vi "UAMatchLabel.vi"(8 "error in (no error)":errorcluster caption="错误输入（无错误）", 11 "String":string) -> (0 "error out":errorcluster caption="错误输出", 3 "keyValues":T1(array[cluster]))   [LabVIEW 2014, in "OPCUA XML(dev).lvlib"]
uses:
  <vilib>/regexp/Match Regular Expression.xnode
  OPCUA XML(dev).lvlib
panel:
  out "Array":string[](array[string])
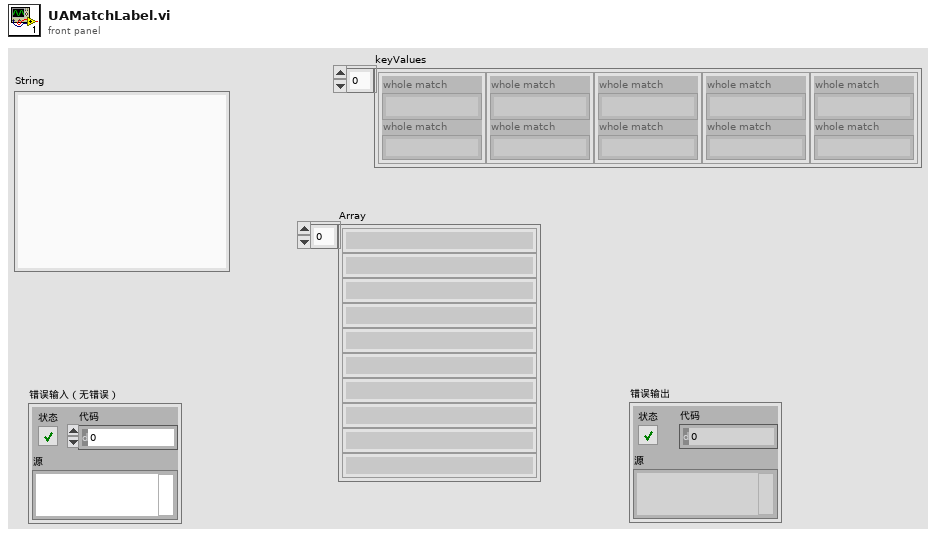
[diagram p1: front panel]
types:
  T1 = cluster{"whole match":string, "whole match":string}[]
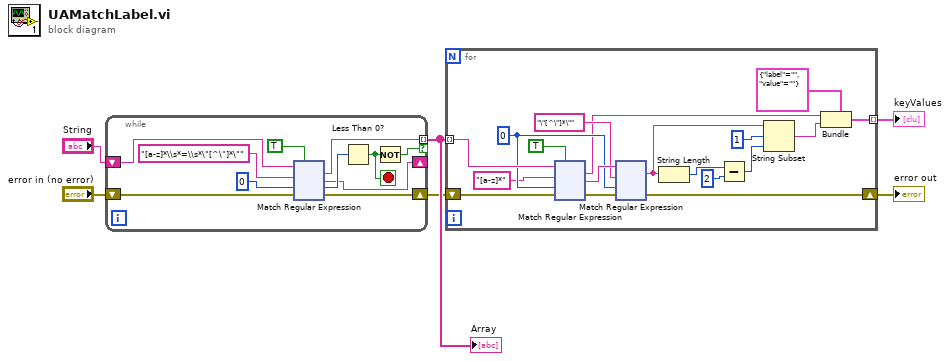
[diagram p0: block diagram]
diagram:
  n1 = while {
    shift-right: [w12] -> _
    shift-left: "String" -> [w17]
    tunnel: [w14] -> w4 mode=indexing if=w7
    shift-right: [w9] -> w3
    shift-left: "error in (no error)" -> [w10]
    stop <- w8 stop-if-true
    n2 = xnode "Match Regular Expression"("input string"=w17, "regular expression"="[a-z]*\\s*=\\s*\"[^\"]*\"", "offset (0)"=0, "error in"=w10, "ignore case? (F)"=TRUE) -> ("whole match"=w14:string, "after match"=w12:string, "offset past match"=w13:i32, "error out"=w9:errorcluster)  [unwired: 1 in, 1 out]
    n3 = Less Than 0?(x=w13) -> (x < 0?=w8:bool)
    n4 = Not(x=w8) -> (.not. x?=w7:bool)
  }
  "Array" <- w4
  n5 = for {
    tunnel: w4 -> [w149] mode=indexing
    shift-right: [w141] -> w2
    shift-left: w3 -> [w143]
    tunnel: [w133] -> w1 mode=indexing
    w145 = 0 ("offset (0)")
    n6 = xnode "Match Regular Expression"("input string"=w149, "regular expression"="[a-z]*", "offset (0)"=w145, "error in"=w143, "ignore case? (F)"=TRUE) -> ("whole match"=w135:string, "after match"=w147:string, "error out"=w142:errorcluster)  [unwired: 1 in, 2 out]
    n7 = xnode "Match Regular Expression"("input string"=w147, "regular expression"="\"[^\"]*\"", "offset (0)"=w145, "error in"=w142) -> ("whole match"=w139:string, "error out"=w141:errorcluster)  [unwired: 2 in, 3 out]
    n8 = String Length(string=w139) -> (length=w137:i32)
    n9 = Subtract(x=w137, y=2) -> (x-y=w138:i32)
    n10 = String Subset(string=w139, offset (0)=1, length (rest)=w138) -> (substring=w134:string)
    n11 = Bundle(cluster=cluster{"label":string, "value":string} {"label"="", "value"=""}, "label"=w135, "value"=w134) -> (w133:cluster{"label":string, "value":string})
  }
  "error out" <- w2
  "keyValues" <- w1
